vi "SECADO_JKI_v120.vi"() -> ()   [LabVIEW 2017]
uses:
  Typedefs/SECADO_datos.Ensayo--Cluster.ctl
  Agilent 34970/34970_Configuracion.ctl
  Typedefs/SECADO_constantes.Ensayo--Cluster.ctl
  Typedefs/SECADO_datos.Lecho--Cluster.ctl
  Typedefs/SECADO_calculos.Ensayo--Cluster.ctl
  Typedefs/SECADO_comms--Cluster.ctl
  MODBUS_EUROTHERM P116_485/numDecimales--Enum.ctl
  Agilent 34970/34970_Module Control.ctl
  Timing/Timing_Module Control.ctl
  File/File_Module Control.ctl
  MODBUS_EUROTHERM P116_485/Eurotherm_2023_Module.ctl
  MODBUS_EUROTHERM P116_485/Address.ctl
  MODBUS_EUROTHERM P116_485/P116x1ch.ctl
  MODBUS_EUROTHERM P116_485/1xP116.ctl
panel:
  out "TEMP_9, C":dbl caption="C" format="%.1f"
  out "TEMP_8, C":dbl caption="C" format="%.1f"
  out "TEMP_7, C":dbl caption="C" format="%.1f"
  out "SET_CAUDAL, g/s":dbl caption="kg/h" format="%.2f"
  out "HUM_EXT, f1":dbl caption="C" format="%.1f"
  out "error out":errorcluster
  in  "Tab Control":T1(tab)
  in  "PRES_EXT, Pa":dbl caption="C" format="%.1f"
  out "Fecha":string
  out "#.datos":i32
  out "Calculos.Ensayo":T2={"Agua.evap, g/s"=0.0, "Hum.lecho, %"=1.0, "Q.aire.seco, W"=50.0, "Q.evaporacion, W"=230.0, "Porosidad"=60.0, "Vel.air.reactor, m/s"=1.0} {"Agua.evap, g/s" format="%.2f"; "Hum.lecho, %" format="%.2f"; "Q.aire.seco, W" format="%.2f"; "Q.evaporacion, W" format="%.2f"; "Porosidad" format="%.2f"; "Vel.air.reactor, m/s" format="%.2f"}
  out "TEMP_EXT, C":dbl caption="C" format="%.1f"
  out "TEMP_6, C":dbl caption="C" format="%.1f"
  out "TEMP_5, C":dbl caption="C" format="%.1f"
  in  "t.wait, ms":dbl=333.0 caption="s"
  in  "but.setpoint":bool
  out "TEMP_R, C":dbl caption="C" format="%.1f"
  out "SET_TEMP_R, C":dbl caption="C" format="%.1f"
  out "TEMP_1, C":dbl caption="C" format="%.1f"
  out "TEMP_2, C":dbl caption="C" format="%.1f"
  out "TEMP_3, C":dbl caption="C" format="%.1f"
  out "TEMP_4, C":dbl caption="C" format="%.1f"
  out "CAUDAL.vol, m³/h":dbl caption="kPa" format="%.2f"
  out "HUM_REL_3, f1":dbl caption="%" format="%.2f"
  out "HUM_REL_4, f1":dbl caption="%" format="%.2f"
  out "CAUDAL, kg/h":dbl caption="kg/h" format="%.2f"
  out "POTENCIA, W":dbl caption="kW" format="%.2f"
  out "Error":bool
  out "t.ensayo, min":dbl caption="C" format="%.1f"
  in  "t.muestreo, s":dbl=10.0 caption="s" format="%.1f"
  in  "but.inicioMedida":bool
  out "Fichero":path
  out "Status":string
  in  "but.finalMedida":bool
  out "Hora":string
  in  "but.Fin":bool
  out "Prog. Running?":bool
  out "Seq. Loaded?":bool
  out "Prog. Aborted?":bool
  out "States History":string caption="Last State"
  out "t.ciclo, s":dbl format="%.1f"
  out "dt.ciclo, s":dbl format="%.1f"
  out "POTENCIA CALEFACCION":cluster{dbl[], dbl[]}[](graph)
  out "CAUDAL":cluster{dbl[], dbl[]}[](graph)
  out "EUROTHERM":cluster{dbl[], dbl[]}[](graph)
  out "Q CEDIDO Y ABSORBIDO":cluster{dbl[], dbl[]}[](graph)
  out "CONCENTRACION HUMEDAD":cluster{dbl[], dbl[]}[](graph)
  out "AGUA EVAPORADA AL AIRE":cluster{dbl[], dbl[]}[](graph)
  out "VELOCIDAD AIRE":cluster{dbl[], dbl[]}[](graph)
  out "TEMPERATURA":cluster{dbl[], dbl[]}[](graph)
  out "HUMEDAD":cluster{dbl[], dbl[]}[](graph)
  out "PRES_DIF":cluster{dbl[], dbl[]}[](graph)
  out "Agilent.configuracion.file":path
  out "Dispositivos":T3=[["Temperatura", "emulsion_entrada", "101", "C", "0.00"], ["Temperatura", "emulsion_salida", "102", "C", "0.00"], ["Temperatura", "agua_entrada", "107", "C", "0.00"], ["Temperatura", "agua_salida", "108", "C", "0.00"], ["Temperatura", "ambiente", "105", "C", "0.00"], ["Presion", "emulsion_entrada", "103", "bar", "0.00"], ["Presion", "emulsion_salida", "109", "bar", "0.00"], ["Presion", "agua_entrada", "110", "bar", "0.00"], ["Presion", "agua_salida", "114", "bar", "0.00"], ["Presion", "", "", "bar", "0.00"], ["Caudal", "caudalimetro", "120", "L/h", "0.00"], ["Caudal", "", "", "L/h", "0.00"], ["Caudal", "", "", "L/h", "0.00"], ["Caudal", "", "", "L/h", "0.00"], ["Caudal", "", "", "L/h", "0.00"]] caption="Agilent.configuracion.canales"
  out "Datos.ensayo":T4 {"Presion.abs.ext, Pa" format="%.2f"; "Temp.termopar.9, C" format="%.2f"; "Temp.termopar.8, C" format="%.2f"; "Temp.termopar.7, C" format="%.2f"; "Porosidad," format="%.2f"; "Vel.air.reactor, m/s" format="%.2f"; "Q.evaporacion, W" format="%.2f"; "Q.aire.seco, W" format="%.2f"; "Humedad.lecho, f1" format="%.2f"; "Temperatura.ext, C" format="%.2f"; "Humedad.Rel.ext, f1" format="%.2f"; "Q.set.caudal, g/s" format="%.2f"; "Temp.termopar.6, C" format="%.2f"; "Temp.termopar.5, C" format="%.2f"; "P116.output, W" format="%.2f"; "Agua.evapor, g/s" format="%.2f"; "Humedad.rel.3, f1" format="%.2f"; "Temp.pt100.4, C" format="%.2f"; "Temp.pt100.3, C" format="%.2f"; "Q.caudal, g/s" format="%.2f"; "Humedad.rel.4, f1" format="%.2f"; "P116.temperatura, C" format="%.2f"; "P116.set.temp, C" format="%.2f"; "P116.output, %" format="%.2f"; "Temp.pt100.2, C" format="%.2f"; "Q.caudal.vol, m3/h" format="%.2f"; "Temp.pt100.1, C" format="%.2f"; "Tiempo (min)" format="%.2f"}
  out "Datos.Lecho":T5={"Clasificacion"="Grueso (2,5<Dp<4", "Masa, g"=500.0, "Altura, cm"=45.0, "Diam_part, mm"=5.0, "Dens_part, g/cm3"=1.0, "Hum_ini, f1"=60.0, "Temp_ini, C"=25.0} {"Hum_ini, f1" format="%.2f"; "Temp_ini, C" format="%.2f"; "Masa, g" format="%.2f"; "Altura, cm" format="%.2f"; "Diam_part, mm" format="%.2f"; "Dens_part, g/cm3" format="%.2f"}
  out "Constantes.Ensayo":T6={"Num.Ensayo"=0, "Diam_reactor, cm"=0.0, "Resistencia, ohm"=50.0, "Voltaje_resist, vac"=0.0, "Hum_ext, f1"=0.0, "Vel.min_fluido, m/s"=0.0, "Vel_arrastre, m/s"=10.0, "SET Caudal_vent, g/s"=0.0} {"Vel_arrastre, m/s" format="%.2f"; "SET Caudal_vent, g/s" format="%.2f"; "Diam_reactor, cm" format="%.2f"; "Resistencia, ohm" format="%.2f"; "Voltaje_resist, vac" format="%.2f"; "Hum_ext, f1" format="%.2f"; "Vel.min_fluido, m/s" format="%.2f"}
  # "Mayo.2025 asslcdms v1.2.0 LV2017"
  # "IMPORTANTE\nAunque configuremos los sensores, estos se leeran directamente por flowbus"
  # "--- SECADO ---"
  # "REACTOR"
  # "Pulsar para cambiar temperatura"
  # "VENTEO"
  # "RESISTENCIA"
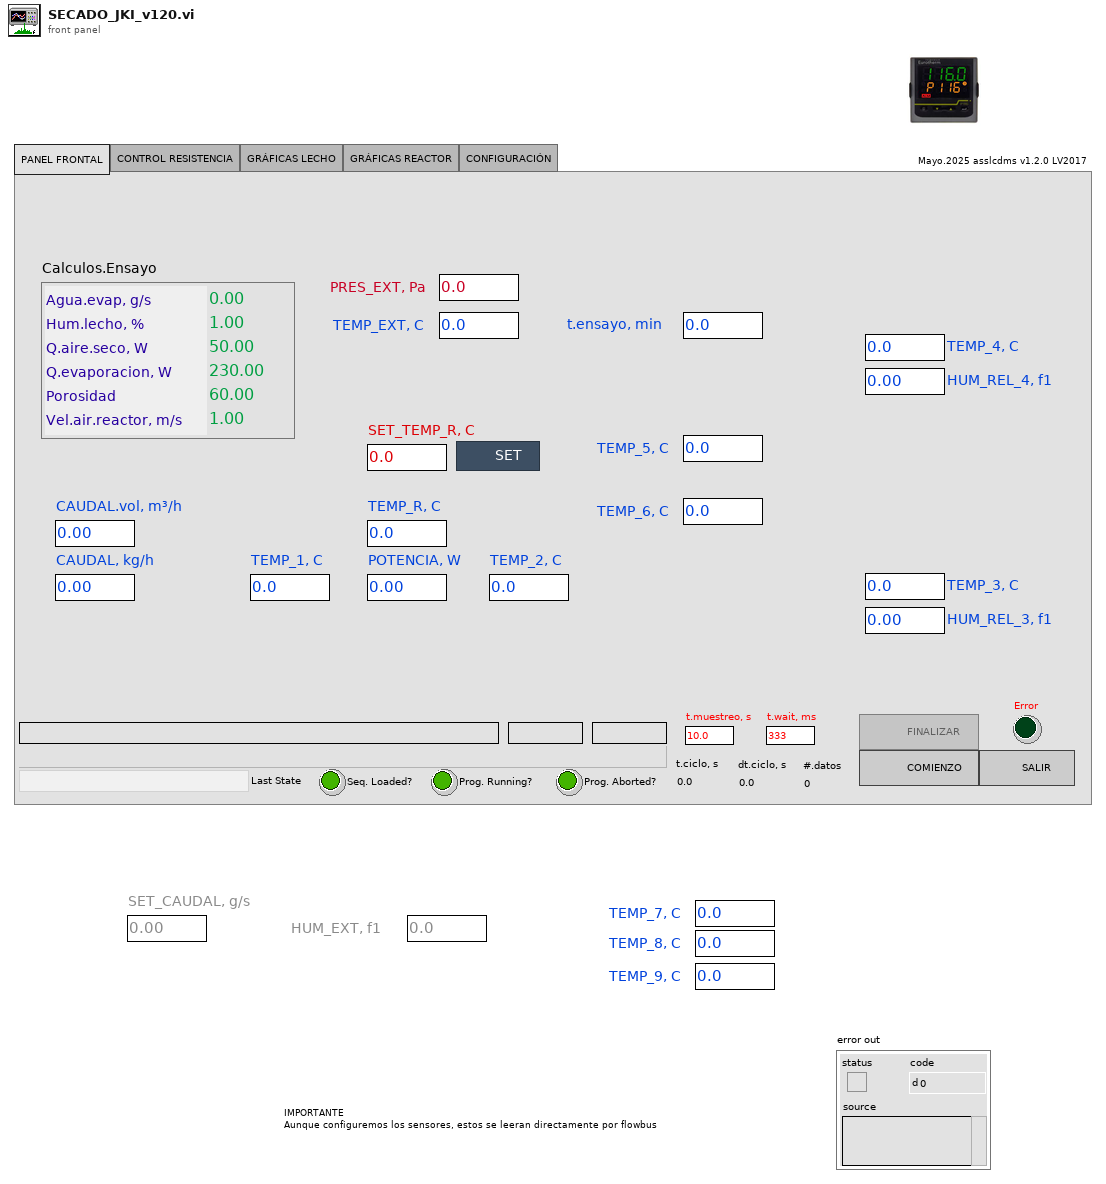
[diagram p1: front panel]
types:
  T1 = enum32{"PANEL FRONTAL", "CONTROL RESISTENCIA", "GRÁFICAS LECHO", "GRÁFICAS REACTOR", "CONFIGURACIÓN"}
  T2 = typedef "SECADO_calculos.Ensayo--Cluster.ctl" = cluster{"Agua.evap, g/s":dbl, "Hum.lecho, %":dbl, "Q.aire.seco, W":dbl, "Q.evaporacion, W":dbl, "Porosidad":dbl, "Vel.air.reactor, m/s":dbl}
  T3 = typedef "34970_Configuracion.ctl" = string[][]
  T4 = typedef "SECADO_datos.Ensayo--Cluster.ctl" = cluster{"Tiempo (min)":dbl, "Temperatura.ext, C":dbl, "Humedad.Rel.ext, f1":dbl, "Temp.pt100.1, C":dbl, "Temp.pt100.2, C":dbl, "Temp.pt100.3, C":dbl, "Temp.pt100.4, C":dbl, "Temp.termopar.5, C":dbl, "Temp.termopar.6, C":dbl, "Humedad.rel.3, f1":dbl, "Humedad.rel.4, f1":dbl, "Q.caudal.vol, m3/h":dbl, "P116.set.temp, C":dbl, "P116.temperatura, C":dbl, "P116.output, %":dbl, "P116.output, W":dbl, "Q.set.caudal, g/s":dbl, "Q.caudal, g/s":dbl, "Agua.evapor, g/s":dbl, "Humedad.lecho, f1":dbl, "Q.aire.seco, W":dbl, "Q.evaporacion, W":dbl, "Porosidad, ":dbl, "Vel.air.reactor, m/s":dbl, "Temp.termopar.7, C":dbl, "Temp.termopar.8, C":dbl, "Temp.termopar.9, C":dbl, "Presion.abs.ext, Pa":dbl}
  T5 = typedef "SECADO_datos.Lecho--Cluster.ctl" = cluster{"Clasificacion":string, "Masa, g":dbl, "Altura, cm":dbl, "Diam_part, mm":dbl, "Dens_part, g/cm3":dbl, "Hum_ini, f1":dbl, "Temp_ini, C":dbl}
  T6 = typedef "SECADO_constantes.Ensayo--Cluster.ctl" = cluster{"Num.Ensayo":i32, "Diam_reactor, cm":dbl, "Resistencia, ohm":dbl, "Voltaje_resist, vac":dbl, "Hum_ext, f1":dbl, "Vel.min_fluido, m/s":dbl, "Vel_arrastre, m/s":dbl, "SET Caudal_vent, g/s":dbl}
  T7 = enum32{"Invalid", "Standard", "Closed", "Hidden", "Minimized", "Maximized"}
  T8 = enum32{"invalid app kind", "Development System", "Run Time System", "Student Edition", "Embedded LabVIEW", "Evaluation", "Custom"}
  T9 = typedef "SECADO_comms--Cluster.ctl" = cluster{"Eurotherm":refnum<visa-resource-name>, "CDT":bool, "Agilent":refnum<visa-resource-name>, "AGL":bool, "#dec":T10}
  T10 = typedef "numDecimales--Enum.ctl" = u16
  T11 = typedef "34970_Module Control.ctl" = enum16{"INICIALIZA", "CONFIGURA CANALES", "LECTURA PT100", "LECTURA TERMOPAR", "LECTURA HUMEDAD", "LECTURA CAUDAL", "SHUTDOWN"}
  T12 = typedef "Timing_Module Control.ctl" = enum16{"Initialize Time", "Check Time"}
  T13 = enum8{"Enabled", "Disabled", "Disabled and Grayed Out"}
  T14 = typedef "File_Module Control.ctl" = enum16{"Initialize", "Save Head", "Save Data", "Shutdown"}
  T15 = typedef "Address.ctl" = enum16{"Add 1", "Add 2", "Add 3", "Add 4", "Add 5", "Add 6", "Add 10", "Add 11", "Add 12", "Add 13"}
  T16 = typedef "Eurotherm_2023_Module.ctl" = enum16{"Initialize", "Write setpoint", "Read data", "Write ramp rate", "Set constante proporcional", "Set constante integral", "Set constante diferencial", "Set ouput limit LOW", "Set ouput limit HIGH", "Shutdown"}
  T17 = typedef "P116x1ch.ctl" = cluster{"TargetSP":T18, "WorkingSP":T18, "Temperatura":T18, "RateSP":T18, "Potencia":T18, "Potencia max":T18}
  T18 = typedef "1xP116.ctl" = cluster{"Ch1":dbl}
  T19 = cluster{"Core":cluster{"Current VI Reference":refnum<vi>, "Close Panel on Exit?":bool}, "datos.Ensayo":T4, "data array":T4[], "nPuntos":i32, "Filename":path, "Comunicaciones":T9, "delta.t.ciclo":dbl, "Status.string":string, "Step.sample.time":dbl, "Step.timeout?":bool, "Prog.running?":bool, "Prog.aborted?":bool, "Seq.loaded?":bool, "#Datos":i32, "Datos.Lecho":T5, "Constantes.Ensayo":T6}
  T20 = cluster{"Current VI Reference":refnum<vi>, "Close Panel on Exit?":bool}
  T21 = cluster{"processVal":dbl, "targetSP":dbl, "workingSP":dbl, "workingOut":dbl}
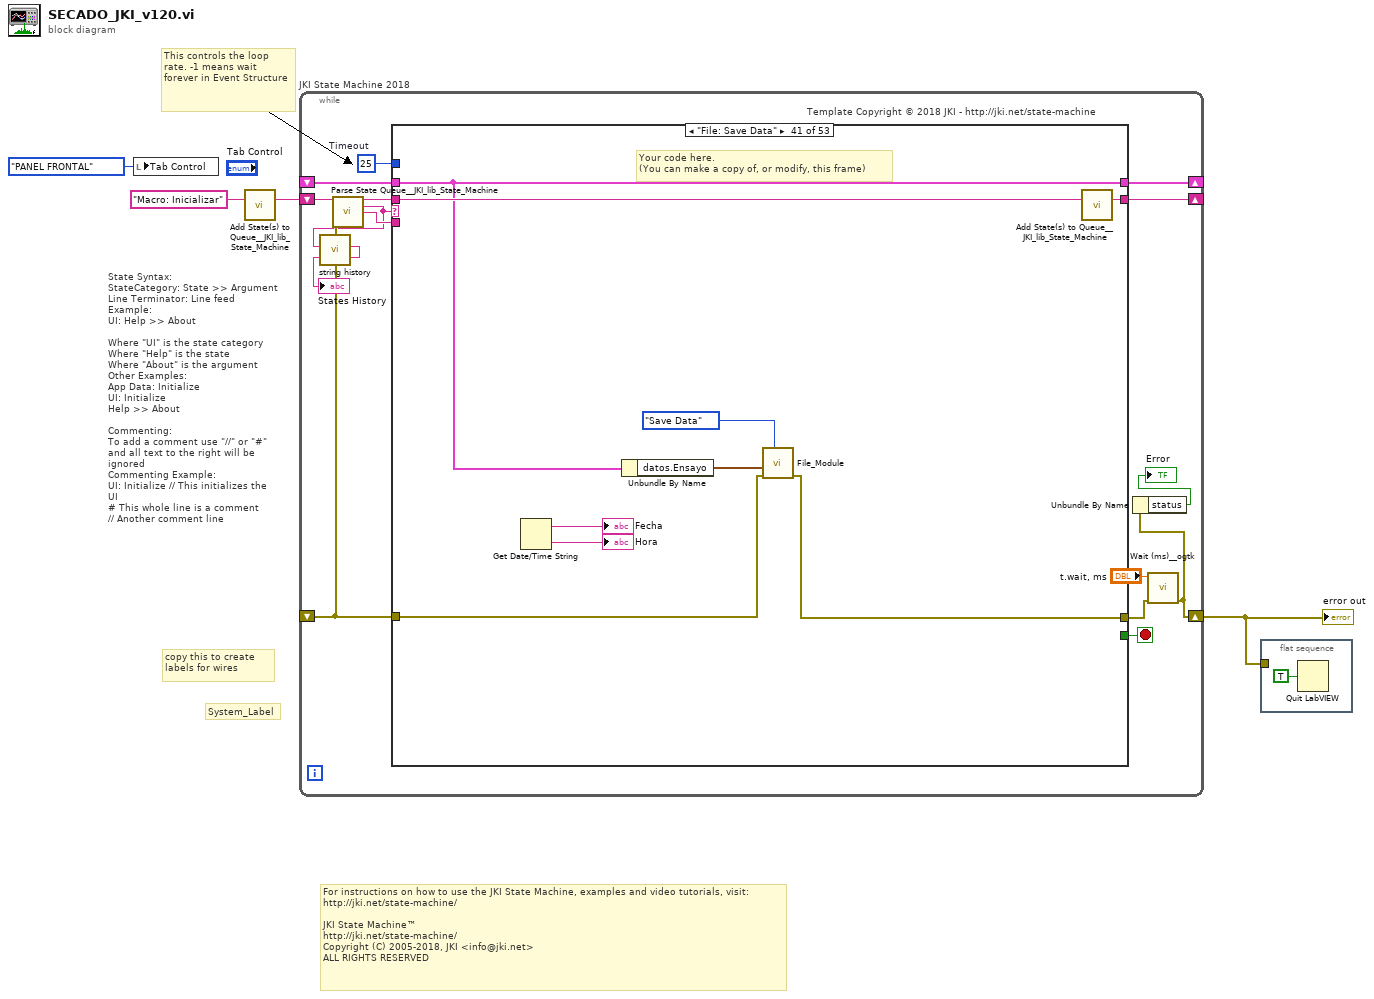
[diagram p0: block diagram]
diagram:
  # "For instructions on how to use the JKI State Machine, examples and video tutorials, visit:\nhttp://jki.net/state-machine/\n\nJKI State Machine™\nhttp://jki.net/state-machine/\nCopyright (C) 2005-2018, JKI <info@jki.net>\nALL RIGHTS RESERVED"
  # "State Syntax:\nStateCategory: State >> Argument\nLine Terminator: Line feed\nExample:\nUI: Help >> About\n\nWhere \"UI\" is the state category\nWhere \"Help\" is the state\nWhere \"About\" is the argument\nOther Examples:\nApp Data: Initialize\nUI: Initialize\nHelp >> About\n\nCommenting:\nTo add a comment use \"//\" or \"#\" and all text to the right will be ignored\nCommenting Example:\nUI: Initialize // This initializes the UI\n# This whole line is a comment\n// Another comment line"
  # "copy this to create labels for wires"
  # "This controls the loop rate. -1 means wait forever in Event Structure"
  # "System_Label"
  n1 = local write "Tab Control"(T1."PANEL FRONTAL" ("Tab Control")) -> ()
  n2 = call <vilib>:"Add State(s) to Queue__JKI_lib_State_Machine.vi"("State(s) in (\"\")"="Macro: Inicializar") -> ("States Out"=w4:string)  [unwired: 14 in]
  n3 = while "JKI State Machine 2018" {
    shift-right: [w14] -> _
    shift-left: _ -> [w13]
    shift-right: [w6] -> w2
    shift-left: _ -> [w11]
    shift-right: [w16] -> _
    shift-left: w4 -> [w17]
    stop <- w15 stop-if-true
    w12 = 25  # Timeout
    # "Template Copyright © 2018 JKI - http://jki.net/state-machine"
    n4 = call <vilib>:"Parse State Queue__JKI_lib_State_Machine.vi"("State Queue"=w17, "Error In (no error)"=w11) -> ("Remaining States"=w19:string, "Current State"=w9:string, "Arguments"=w18:string)  [unwired: 11 in]
    n5 = call "string history.vi"("State Queue"=w9) -> ("State Queue history (last on top)"=→"States History":string)  [unwired: 10 in]
    n6 = case shown="\"File: Save Data\"" w9 {
      selector: w9 -> [_ _ w61 _ _ _ _ _ _ _ _ _ _ _ _ _ _ _ _ _ _ _ _ _ _ _ _ _ _ _ _ _ _ _ _ _ _ _ _ _ _ _ _ _ _ _ _ _ _ _ _ _ _]
      tunnel: w19 -> [w26 w60 w65 w84 w90 w95 w99 w119 w135 w141 w145 w152 w163 w171 w175 w179 w183 w189 w201 w209 w221 w225 w229 w235 w246 w319 w329 w358 w427 w455 w465 w475 _ w493 w498 w503 w508 w519 w523 w535 w544 w548 w556 w560 w574 w590 w601 w613 w640 w644 w661 w665 w684]
      tunnel: w18 -> [_ _ _ _ _ _ _ _ _ _ _ _ _ _ _ _ _ _ _ _ _ _ _ w230 w240 _ _ _ _ _ _ _ _ _ _ _ _ _ _ _ _ _ _ _ _ _ _ _ _ _ _ _ _]
      tunnel: w13 -> [w24 w57 w63 w77 w87 w93 w96 _ w132 w136 w142 w150 w159 w167 w173 w177 w180 w187 w191 w207 w219 w222 w227 w233 w242 w315 w321 w342 w366 w452 w457 w472 w480 w489 w495 w500 w505 w516 w520 w533 w538 w545 w554 w557 w563 w581 w595 w606 w637 w641 w654 w662 w679]
      tunnel: [w23 w58 w67 w81 errorcluster {"status"=FALSE, "code"=0, "source"=""} ("error out") w92 w97 w116 w133 w137 w143 w148 w160 w168 w172 w176 w181 w184 w197 w205 w217 w223 w226 w231 w243 w316 w327 w345 w383 w453 w463 w473 w484 w491 w496 w501 w506 w517 w521 w529 w540 w546 w551 w558 w565 w583 w597 w608 w634 w642 w649 w663 w680] -> w8
      tunnel: w11 -> [w22 w58 w66 w81 w86 w92 w97 w116 w133 w138 w143 w149 w154 w164 w172 w176 w181 w185 w198 w206 w218 w223 w226 w232 w244 w316 w327 w345 w383 w453 w463 w473 w484 w491 w496 w501 w506 w517 w521 w530 w541 w546 w551 w558 w564 w582 w596 w607 w636 w642 w655 w663 w681]
      tunnel: [w25 w59 w64 w83 w89 w94 w98 w118 w134 w140 w144 w151 w162 w170 w174 w178 w182 w188 w200 w208 w220 w224 w228 w234 w245 w318 w328 w357 w426 w454 w464 w474 w485 w492 w497 w502 w507 w518 w522 w534 w543 w547 w555 w559 w573 w589 w600 w612 w639 w643 w660 w664 w683] -> w16
      tunnel: [_ _ _ _ _ TRUE _ _ _ _ _ _ _ _ _ _ _ _ _ _ _ _ _ _ _ _ _ _ _ _ _ _ _ _ _ _ _ _ _ _ _ _ _ _ _ _ _ _ _ _ _ _ _] -> w15
      tunnel: [w21 w57 w63 w82 w87 w93 w96 w117 w131 w136 w142 w147 w159 w167 w173 w177 w180 w187 w196 w203 w214 w222 w227 w233 w242 w315 w321 w342 w408 w452 w456 w470 w479 w488 w495 w500 w505 w516 w520 w528 w538 w545 w554 w557 w570 w587 w599 w611 w633 w641 w654 w662 w682] -> w14
      tunnel: w12 -> [w20 _ _ _ _ _ _ _ _ _ _ _ _ _ _ _ _ _ _ _ _ _ _ _ _ _ _ _ _ _ _ _ _ _ _ _ _ _ _ _ _ _ _ _ _ _ _ _ _ _ _ _ _]
      frame "", "Event Structure", "Idle" {
        # "executes when the state queue is empty"
        n7 = event shown="[4] \"but.finalMedida\": Value Change" {
          selector: _ -> [_ _ _ _ _ _]
          dyn-events: _ -> [_ _ _ _ _ _]
          timeout: w20 -> [_ _ _ _ _ _]
          tunnel: w26 -> [w30 w35 w40 w45 w50 w56]
          tunnel: [w29 w34 w39 w44 w49 w55] -> w25
          tunnel: w24 -> [w27 w32 w37 w42 w47 w53]
          tunnel: [w28 w33 w38 w43 w48 w54] -> w23
          tunnel: w22 -> [w28 w33 w38 w43 w48 w54]
          tunnel: [w27 w32 w37 w42 w47 w53] -> w21
          event Timeout {
            # "README FIRST\nThis VI template should be used by dragging & dropping it from the Functions palette onto the Block Diagram of a new, blank VI, which will place it's contents into the blank VI.\n\nDo not edit the VI found in the palette.  Only edit the state machine after it is placed into your blank VI.\n\nFor instructions on how to use the JKI State Machine, examples and video tutorials, visit:\nhttp://jki.net/state-machine/\n\nDELETE THIS NOTE AFTER READING"
            # "Timeout Frame\n(this will only execute if the Event Structure timeout is >= 0)"
            n8 = event-data() -> ()  [unwired: 1 in, 1 out]
            n9 = call <vilib>:"Add State(s) to Queue__JKI_lib_State_Machine.vi"("State(s) in (\"\")"=w30) -> ("States Out"=w29:string)  [unwired: 14 in]
          }
          event "but.Fin": Value Change {
            # "Exit Button Value Change (pressed) Event\n(this executes Macro: Exit to terminate the VI)"
            n10 = event-data() -> ()  [unwired: 1 in, 1 out]
            n11 = call <vilib>:"Add State(s) to Queue__JKI_lib_State_Machine.vi"("State(s) in Front (\"\")"="Macro: Exit", "State(s) in (\"\")"=w35) -> ("States Out"=w34:string)  [unwired: 13 in]
          }
          event "but.setpoint": Value Change {
            # "Set Button Value Change (pressed) Event\n(this executes Macro: Change settings to change SP)"
            n12 = event-data() -> ()  [unwired: 1 in, 6 out]
            n13 = call <vilib>:"Add State(s) to Queue__JKI_lib_State_Machine.vi"("State(s) in Front (\"\")"="Change settings: Eurotherm temp", "State(s) in (\"\")"=w40) -> ("States Out"=w39:string)  [unwired: 13 in]
          }
          event "but.inicioMedida": Value Change {
            # "Button Inicio.Medida (pressed) Event\n(this executes Macro: Run Measure)"
            n14 = event-data() -> ()  [unwired: 1 in, 6 out]
            n15 = call <vilib>:"Add State(s) to Queue__JKI_lib_State_Machine.vi"("State(s) in Front (\"\")"="Macro: Run Measure", "State(s) in (\"\")"=w45) -> ("States Out"=w44:string)  [unwired: 13 in]
          }
          event "but.finalMedida": Value Change {
            # "Set Button Value Change (pressed) Event\n(this executes Macro: Change settings to change SP)"
            n16 = event-data() -> ()  [unwired: 1 in, 6 out]
            n17 = call <vilib>:"Add State(s) to Queue__JKI_lib_State_Machine.vi"("State(s) in Front (\"\")"="Macro: Abort Measure", "State(s) in (\"\")"=w50) -> ("States Out"=w49:string)  [unwired: 13 in]
          }
          event Panel Close? {
            # "Discard the event because we'll close the front panel ourselves in Macro: Exit"
            # "Close Panel button (pressed) Event\n(this executes Macro: Exit to terminate the VI)"
            n18 = event-data() -> ()  [unwired: 1 in, 1 out]
            n19 = event-data("Discard?"=TRUE) -> ()  [unwired: 1 in, 1 out]
            n20 = call <vilib>:"Add State(s) to Queue__JKI_lib_State_Machine.vi"("State(s) in Front (\"\")"="Macro: Exit", "State(s) in (\"\")"=w56) -> ("States Out"=w55:string)  [unwired: 13 in]
          }
        }
      }
      frame "---------- Core ----------" {
        # "Do not put any code in this frame.\n(it is a separator no-op)"
        n21 = call <vilib>:"Add State(s) to Queue__JKI_lib_State_Machine.vi"("State(s) in (\"\")"=w60) -> ("States Out"=w59:string)  [unwired: 14 in]
      }
      frame Default {
        w70 = 42 items=["No error", "Argument error", "Memory is full", "Out of zone", "End of file", "File already open", "Generic file I/O error", "File not found", "File permission error", "Disk is full", "Duplicate path", "Too many files open", "System feature not enabled", "Resource file not found", "Cannot add resource", "Resource not found", "Image not found", "Image memory error", "Pen does not exist", "Config type invalid", "Config token not found", "Config parse error", "Config memory error", "Bad external code format", "Bad external code offset", "External code not present", "Null window", "Destroy window error", "Null menu", "Print aborted", "Bad print record", "Print driver error", "Windows error during printing", "Memory error during printing", "Print dialog error", "Generic print error", "Invalid device refnum", "Device not found", "Device parameter error", "Device unit error", "Cannot open device", "Device call aborted", "Generic error", "Cancelled by user", "Object ID too low", "Object ID too high", "Object not in heap", "Unknown heap", "Unknown object (invalid DefProc)", "Unknown object (DefProc not in table)", "Message out of range", "Invalid (null) method", "Unknown message", "Manager call not supported", "Bad address", "Network operation in progress", "Network operation timed out", "Connection is busy", "Network attribute not supported", "Network error", "Address in use", "System out of memory", "Connection aborted", "Connection refused", "Not connected", "Already connected", "Connection closed", "Initialization error (interapplication manager)", "Bad occurrence", "Wait on unbound occurrence handler", "Occurrence queue overflow", "Datalog type conflict", "Unused", "Unrecognized type (interapplication manager)", "Memory corrupt", "Failed to make temporary DLL", "Old CIN version", "Drag socket not found", "Failed to load drop-object", "Failed to register OLE object", "Failed to release OLE object", "Format specifier type mismatch", "Unknown format specifier", "Too few format specifiers", "Too many format specifiers", "Scan failed", "Newer CIN version", "Error converting to variant", "Runtime menu error", "Password tampered", "Variant attribute not found", "Incompatible variant data type", "Event data is not available", "Event Store is not present", "Occurrence is not found", "Event Queue is not created", "Event info is not available", "Refnum passed is NULL", "Error retrieving Class GUID", "Error retrieving CoClass GUID", "Error retrieving TypeLib GUID.", "Bad built application magic bytes.", "Specific driver is different from the specific driver associated with the Logical Name.", "There is no session opened to the class driver.", "Max Error", "MAX - Error with config objects", "MAX - Error loading configuration", "MAX - Group not supported"]
        # "Current State"
        # "Do not delete, rename, or modify this frame.\n(this is used to capture unhandled states and typos)"
        # "Handle mistyped state name (developer tool)"
        n22 = Format Into String(format string="Software Exception: Unhandled State \"%s\"." ("message"), error in=w66, w61) -> (resulting string=w69:string, error out=w68:errorcluster)  [unwired: 1 in]
        n23 = call <vilib>:"Error Cluster From Error Code.vi"("show call chain? (False)"=TRUE, "error in (no error)"=w68, "error message (\"\")"=w69, "error code (0)"=w70) -> ("error out"=w67:errorcluster)  [unwired: 5 in]
        n24 = call <vilib>:"Add State(s) to Queue__JKI_lib_State_Machine.vi"("State(s) in (\"\")"=w65) -> ("States Out"=w64:string)  [unwired: 14 in]
      }
      frame "Initialize Core Data" {
        # "Do not delete, rename, or modify this frame.\n(this is used to determine panel behavior on exit)"
        # "originally closed?"
        # "exe?"
        # "If panel starts closed or is an EXE, then close it when we exit"
        n25 = property class="VI"() -> ("FP.State"=w74:T7)  [unwired: 2 in, 2 out]
        n26 = property class="App"() -> ("App.Kind"=w80:T8)  [unwired: 2 in, 2 out]
        n27 = control-ref of="Current VI Reference"() -> (w75:refnum<vi>)
        n28 = Equal?(x=w74, y=T7."Closed" ("Front Panel Window:State")) -> (x = y?=w72:bool)
        n29 = Equal?(x=w80, y=T8."Run Time System" ("Application:Kind")) -> (x = y?=w78:bool)
        n30 = Or(x=w72, y=w78) -> (x .or. y?=w76:bool)
        n31 = Bundle By Name(cluster=w77, "Core.Current VI Reference"=w75, "Core.Close Panel on Exit?"=w76) -> (w82:T19)
        n32 = call <vilib>:"Add State(s) to Queue__JKI_lib_State_Machine.vi"("State(s) in (\"\")"=w84) -> ("States Out"=w83:string)  [unwired: 14 in]
      }
      frame "Error Handler" {
        # "Unhandled Error -- Display it"
        # "Handle any errors here.\nYou can also output any states to clean-up after errors occur"
        # "Clear error"
        n33 = call <vilib>:"General Error Handler.vi"("error in (no error)"=w86) -> ()  [unwired: 10 in, 5 out]
        n34 = call <vilib>:"Add State(s) to Queue__JKI_lib_State_Machine.vi"("State(s) in Front (\"\")"="/* Post Error States", "State(s) in (\"\")"=w90) -> ("States Out"=w89:string)  [unwired: 13 in]
      }
      frame "Exit" {
        # "Do not put any code in this frame.\n(No errors that occur here will be handled.)"
        n35 = call <vilib>:"Add State(s) to Queue__JKI_lib_State_Machine.vi"("State(s) in (\"\")"=w95) -> ("States Out"=w94:string)  [unwired: 14 in]
      }
      frame "---------- Data ----------" {
        # "Do not put any code in this frame.\n(It is a separator no-op. You can make a copy of this frame to create a new Data frame)"
        n36 = call <vilib>:"Add State(s) to Queue__JKI_lib_State_Machine.vi"("State(s) in (\"\")"=w99) -> ("States Out"=w98:string)  [unwired: 14 in]
      }
      frame "Data: Initialize" {
        w101 = T6 {"Num.Ensayo"=0, "Diam_reactor, cm"=0.0, "Resistencia, ohm"=50.0, "Voltaje_resist, vac"=0.0, "Hum_ext, f1"=0.0, "Vel.min_fluido, m/s"=0.0, "Vel_arrastre, m/s"=10.0, "SET Caudal_vent, g/s"=0.0}  # Constantes.Ensayo
        w102 = T5 {"Clasificacion"="Grueso (2,5<Dp<4", "Masa, g"=500.0, "Altura, cm"=45.0, "Diam_part, mm"=5.0, "Dens_part, g/cm3"=1.0, "Hum_ini, f1"=60.0, "Temp_ini, C"=25.0}  # Datos.Lecho
        w103 = 0  # #Datos
        w110 = T4 {"Tiempo (min)"=0.0, "Temperatura.ext, C"=0.0, "Humedad.Rel.ext, f1"=0.0, "Temp.pt100.1, C"=0.0, "Temp.pt100.2, C"=0.0, "Temp.pt100.3, C"=0.0, "Temp.pt100.4, C"=0.0, "Temp.termopar.5, C"=0.0, "Temp.termopar.6, C"=0.0, "Humedad.rel.3, f1"=0.0, "Humedad.rel.4, f1"=0.0, "Q.caudal.vol, m3/h"=0.0, "P116.set.temp, C"=0.0, "P116.temperatura, C"=0.0, "P116.output, %"=0.0, "P116.output, W"=0.0, "Q.set.caudal, g/s"=0.0, "Q.caudal, g/s"=0.0, "Agua.evapor, g/s"=0.0, "Humedad.lecho, f1"=0.0, "Q.aire.seco, W"=0.0, "Q.evaporacion, W"=0.0, "Porosidad, "=0.0, "Vel.air.reactor, m/s"=0.0, "Temp.termopar.7, C"=0.0, "Temp.termopar.8, C"=0.0, "Temp.termopar.9, C"=0.0, "Presion.abs.ext, Pa"=0.0}  # datos.Ensayo
        w105 = FALSE  # Prog.aborted?
        w106 = FALSE  # Prog.running?
        w104 = FALSE  # Seq.loaded?
        w108 = 0.0  # Step.sample.time
        w111 = 0.0  # delta.t.ciclo
        w112 = 3600  # nPuntos
